vi "CRYextision level.vi"(6 "measured SPL":dbl[](array[numeric]), 7 "measured frequency":dbl[](array[numeric])) -> (5 "extition level":dbl[](array[numeric]))   [LabVIEW 2013]
panel:
  out "extition level 2":dbl[](array[numeric])
  out "repeated nuber":dbl[](array[numeric])
  in  "delta":dbl[](array[numeric])
  in  "fixed frequency":dbl[](array[numeric])
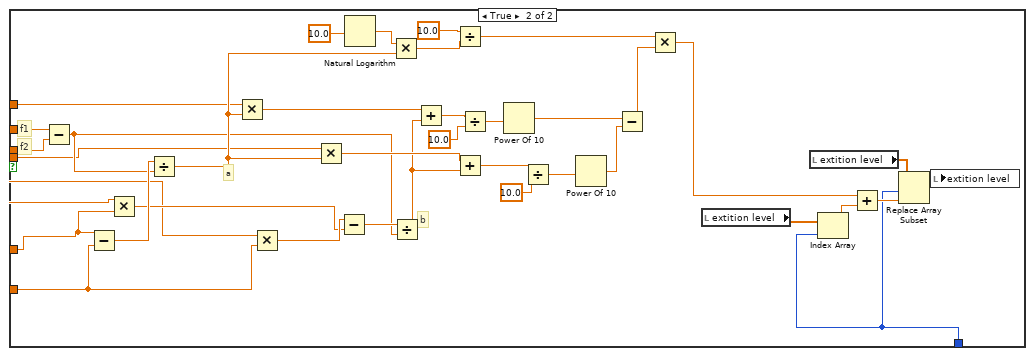
[diagram p4: hidden frame]
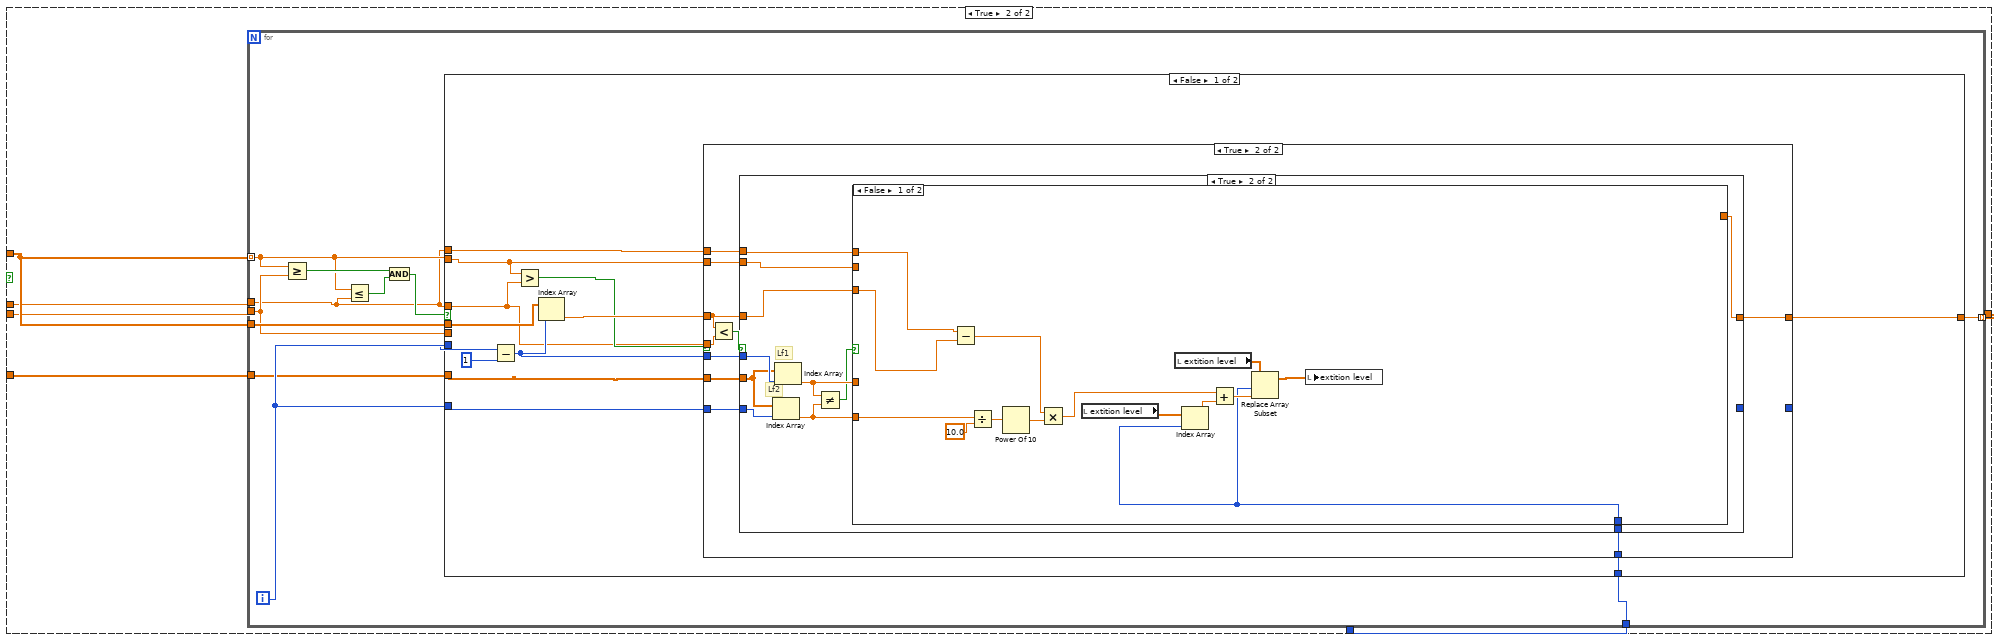
[diagram p5: hidden frame]
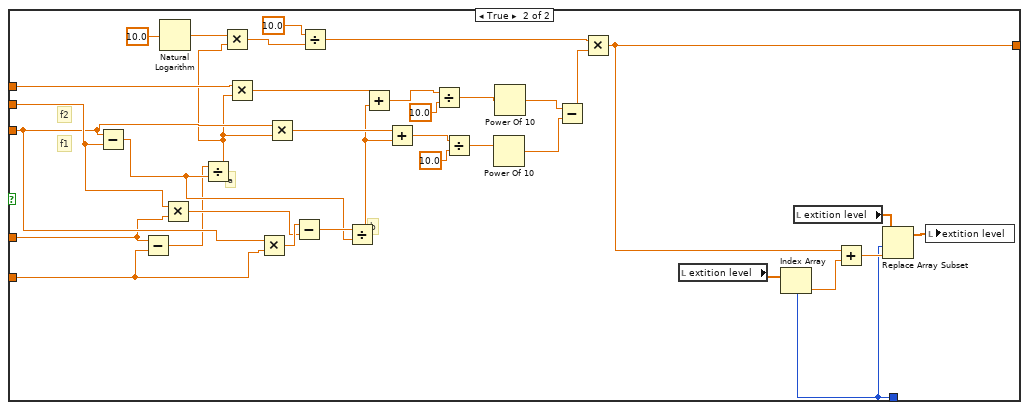
[diagram p8: hidden frame]
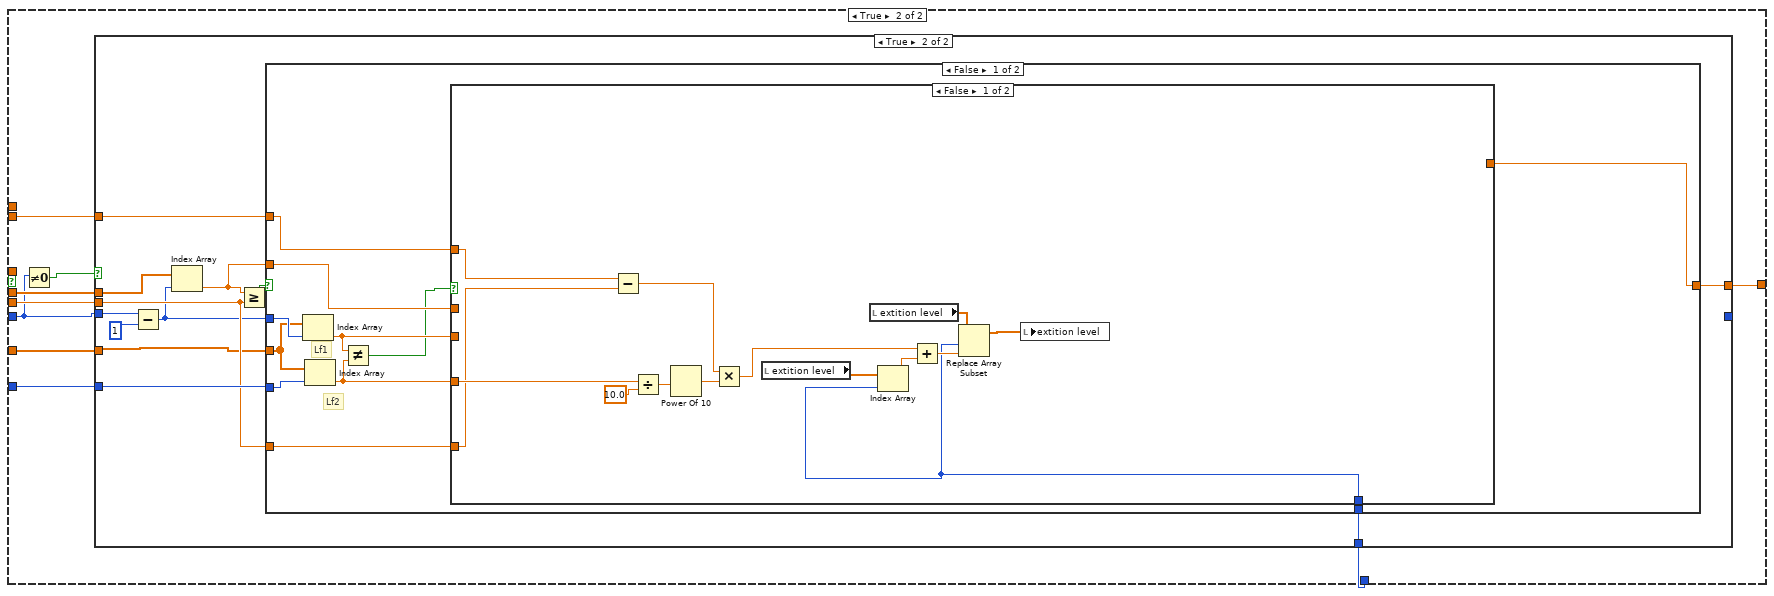
[diagram p9: hidden frame]
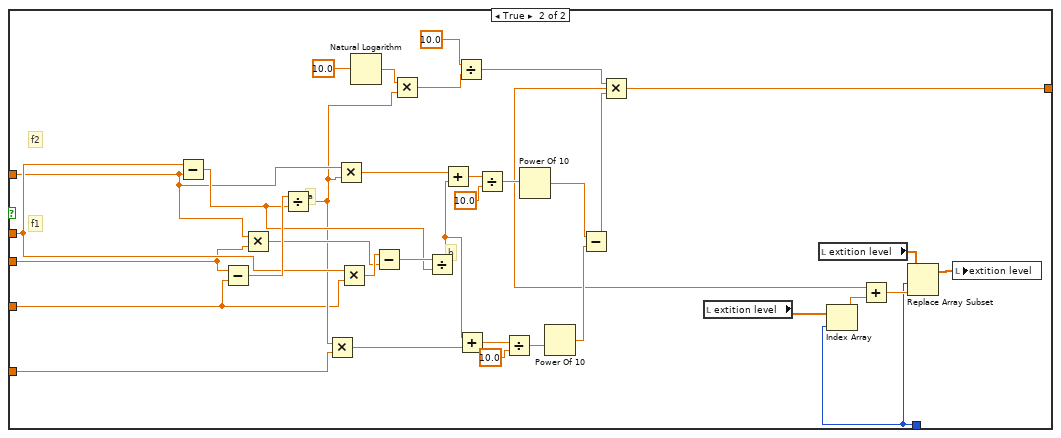
[diagram p11: hidden frame]
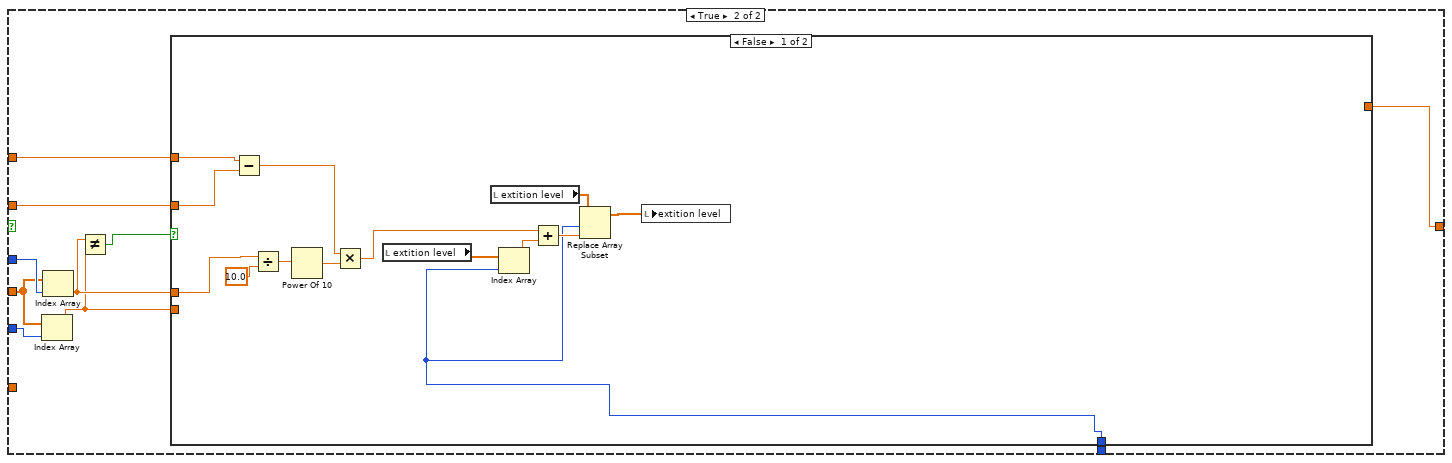
[diagram p12: hidden frame]
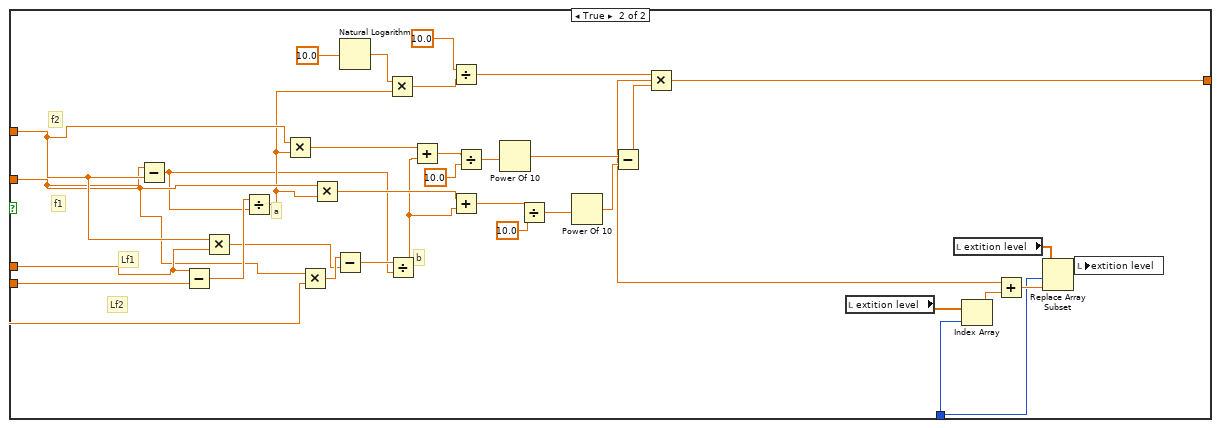
[diagram p13: hidden frame]
diagram:
  n1 = flat-sequence {
    tunnel: [w5] -> w2
    frame #0 {
      n2 = Initialize Array(0.0, 29) -> (w5:dbl[])
      n3 = local write "repeated nuber"(w5) -> ()
      n4 = local write "fixed frequency"(dbl[] [20.0, 25.0, 31.5, 40.0, 50.0, 63.0, 80.0, 100.0, 125.0, 160.0, 200.0, 267.0, 339.0, 436.0, 552.0, 707.7, 899.5, 1112.0, 1406.0, 1827.58, 2288.5, 2813.46, 3501.8, 4289.16, 5099.67, 6148.1, 7303.7, 8309.5, 9452.87, 15500.0]) -> ()
      n5 = local write "extition level"(w5) -> ()
      n6 = local write "delta"(dbl[] [5.0, 6.5, 8.5, 10.0, 13.0, 17.0, 20.0, 25.0, 35.0, 40.0, 67.0, 72.0, 97.0, 116.0, 155.7, 191.8, 202.5, 294.0, 421.58, 460.9, 524.9, 688.3, 787.3, 810.5, 1048.4, 1155.6, 1005.8, 1143.37, 6047.13]) -> ()
    }
  }
  n7 = flat-sequence {
    tunnel: w2 -> [_]
    tunnel: [w8] -> w1
    frame #0 {
      n8 = local read "measured frequency"() -> (w9:dbl[])
      n9 = local read "fixed frequency"() -> (w10:dbl[])
      n10 = for {
        tunnel: w10 -> [w17] mode=indexing
        tunnel: w9 -> [w18]
        tunnel: w10 -> [w16]
        tunnel: [w11] -> w8 mode=indexing
        i -> [w12]
        n11 = Add(x=1.0, y=w12) -> (x+y=w14:dbl)
        n12 = Index Array(array=w16, index=w14) -> (element=w13:dbl)
        n13 = for {
          tunnel: w18 -> [w19] mode=indexing
          tunnel: w17 -> [w26]
          tunnel: w13 -> [w20]
          tunnel: w12 -> [w22]
          tunnel: [w21] -> w11 mode=indexing
          n14 = Greater Or Equal?(x=w19, y=w26) -> (x >= y?=w24:bool)
          n15 = Less Or Equal?(x=w19, y=w20) -> (x <= y?=w25:bool)
          n16 = And(x=w25, y=w24) -> (x .and. y?=w23:bool)
          n17 = case shown="True" w23 {
            tunnel: w22 -> [w27 w31]
            tunnel: [w27 _] -> w21
            frame False {
            }
            frame True {
              n18 = local read "repeated nuber"() -> (w32:dbl[])
              n19 = local read "repeated nuber"() -> (w34:dbl[])
              n20 = Index Array(array=w32, index=w31) -> (element=w30:dbl)
              n21 = Add(x=1.0, y=w30) -> (x+y=w28:dbl)
              n22 = Replace Array Subset(array=w34, new element=w28, index=w31) -> (w33:dbl[])
              n23 = local write "repeated nuber"(w33) -> ()
            }
          }
        }
      }
    }
  }
  n24 = flat-sequence {
    tunnel: w1 -> [_]
    frame #0 {
      n25 = local read "measured frequency"() -> (w36:dbl[])
      n26 = local read "fixed frequency"() -> (w37:dbl[])
      n27 = local read "repeated nuber"() -> (w39:dbl[])
      n28 = local read "measured SPL"() -> (w35:dbl[])
      n29 = local read "delta"() -> (w38:dbl[])
      n30 = for {
        tunnel: w39 -> [w45] mode=indexing
        tunnel: w37 -> [w50] mode=indexing
        tunnel: w38 -> [w41] mode=indexing
        tunnel: w37 -> [w49]
        tunnel: w36 -> [w44]
        tunnel: w35 -> [w43]
        i -> [w40]
        n31 = Add(x=w40, y=1) -> (x+y=w46:i32)
        n32 = Index Array(array=w49, index=w46) -> (element=w48:dbl)
        n33 = Not Equal To 0?(x=w45) -> (x != 0?=w51:bool)
        n34 = case shown="False" w51 {
          tunnel: w44 -> [w66 w147]
          tunnel: w50 -> [w64 w146]
          tunnel: w43 -> [w65 w145]
          tunnel: w48 -> [w63 w144]
          tunnel: [_ w143] -> w42
          tunnel: w40 -> [w62 w142]
          frame False {
            n35 = for {
              tunnel: w66 -> [w74] mode=indexing
              tunnel: w64 -> [w68]
              tunnel: w66 -> [w79]
              tunnel: w65 -> [w73]
              tunnel: w63 -> [w70]
              tunnel: w62 -> [w69]
              tunnel: w63 -> [w67]
              i -> [w71]
              n36 = Add(x=1, y=w71) -> (x+y=w72:i32)
              n37 = Less?(x=w74, y=w68) -> (x < y?=w78:bool)
              n38 = Index Array(array=w79, index=w72) -> (element=w75:dbl)
              n39 = Greater?(x=w75, y=w67) -> (0:w77:bool)
              n40 = And(x=w78, y=w77) -> (x .and. y?=w76:bool)
              n41 = case shown="True" w76 {
                tunnel: w75 -> [_ w91]
                tunnel: w74 -> [_ w85]
                tunnel: w73 -> [_ w90]
                tunnel: w72 -> [_ w89]
                tunnel: w71 -> [_ w88]
                tunnel: w70 -> [_ w87]
                tunnel: w69 -> [_ w86]
                tunnel: w68 -> [_ w84]
                frame False {
                }
                frame True {
                  # "Lf2"
                  # "Lf1"
                  n42 = Index Array(array=w90, index=w88) -> (element=w83:dbl)
                  n43 = Index Array(array=w90, index=w89) -> (element=w82:dbl)
                  n44 = Not Equal?(x=w83, y=w82) -> (x != y?=w81:bool)
                  n45 = case shown="False" w81 {
                    tunnel: w91 -> [_ w113]
                    tunnel: w87 -> [w94 w112]
                    tunnel: w86 -> [w92 w111]
                    tunnel: w85 -> [_ w110]
                    tunnel: w84 -> [w93 w109]
                    tunnel: w83 -> [w95 w107]
                    tunnel: w82 -> [_ w106]
                    frame False {
                      n46 = Subtract(x=w94, y=w93) -> (x-y=w102:dbl)
                      n47 = Divide(x=w95, y=10.0) -> (x/y=w104:dbl)
                      n48 = Power Of 10(x=w104) -> (10^x=w103:dbl)
                      n49 = Multiply(x=w102, y=w103) -> (x*y=w96:dbl)
                      n50 = local read "extition level"() -> (w100:dbl[])
                      n51 = local read "extition level"() -> (w101:dbl[])
                      n52 = Index Array(array=w100, index=w92) -> (element=w99:dbl)
                      n53 = Add(x=w96, y=w99) -> (x+y=w98:dbl)
                      n54 = Replace Array Subset(array=w101, new element=w98, index=w92) -> (w97:dbl[])
                      n55 = local write "extition level"(w97) -> ()
                    }
                    frame True {
                      # "b"
                      # "a"
                      # "f2"
                      # "f1"
                      n56 = Subtract(x=w110, y=w113) -> (x-y=w114:dbl)
                      n57 = Subtract(x=w107, y=w106) -> (x-y=w141:dbl)
                      n58 = Multiply(x=w113, y=w107) -> (x*y=w139:dbl)
                      n59 = Divide(x=w141, y=w114) -> (x/y=w119:dbl)
                      n60 = Multiply(x=w112, y=w119) -> (x*y=w132:dbl)
                      n61 = Multiply(x=w110, y=w106) -> (x*y=w140:dbl)
                      n62 = Multiply(x=w109, y=w119) -> (x*y=w128:dbl)
                      n63 = Subtract(x=w140, y=w139) -> (x-y=w138:dbl)
                      n64 = Natural Logarithm(1:10.0) -> (0:w120:dbl)
                      n65 = Multiply(x=w120, y=w119) -> (x*y=w118:dbl)
                      n66 = Divide(x=w138, y=w114) -> (x/y=w127:dbl)
                      n67 = Add(x=w132, y=w127) -> (x+y=w131:dbl)
                      n68 = Divide(x=10.0, y=w118) -> (x/y=w116:dbl)
                      n69 = Add(x=w128, y=w127) -> (x+y=w124:dbl)
                      n70 = Divide(x=w131, y=10.0) -> (x/y=w129:dbl)
                      n71 = Power Of 10(x=w129) -> (10^x=w123:dbl)
                      n72 = Divide(x=w124, y=10.0) -> (x/y=w126:dbl)
                      n73 = Power Of 10(x=w126) -> (10^x=w122:dbl)
                      n74 = Subtract(x=w123, y=w122) -> (x-y=w115:dbl)
                      n75 = Multiply(x=w116, y=w115) -> (x*y=w108:dbl)
                      n76 = local read "extition level"() -> (w135:dbl[])
                      n77 = local read "extition level"() -> (w136:dbl[])
                      n78 = Index Array(array=w135, index=w111) -> (element=w134:dbl)
                      n79 = Add(x=w108, y=w134) -> (x+y=w133:dbl)
                      n80 = Replace Array Subset(array=w136, new element=w133, index=w111) -> (w137:dbl[])
                      n81 = local write "extition level"(w137) -> ()
                    }
                  }
                }
              }
            }
          }
          frame True {
            n82 = for {
              tunnel: w147 -> [w152] mode=indexing
              tunnel: w146 -> [w153]
              tunnel: w147 -> [w155]
              tunnel: w145 -> [w150]
              tunnel: w142 -> [w154]
              tunnel: [w149] -> w143 mode=indexing
              tunnel: w144 -> [w148]
              i -> [w151]
              n83 = Greater Or Equal?(x=w152, y=w153) -> (x >= y?=w157:bool)
              n84 = Less Or Equal?(x=w152, y=w148) -> (x <= y?=w158:bool)
              n85 = And(x=w157, y=w158) -> (x .and. y?=w156:bool)
              n86 = case shown="False" w156 {
                tunnel: w151 -> [w170 w245]
                tunnel: w155 -> [w171 w247]
                tunnel: w153 -> [_ w248]
                tunnel: w150 -> [w162 w252]
                tunnel: w151 -> [w168 w251]
                tunnel: w152 -> [w161 w250]
                tunnel: w154 -> [w166 w249]
                tunnel: w148 -> [w167 _]
                tunnel: w148 -> [w159 _]
                tunnel: [w163 w244] -> w149
                frame False {
                  n87 = Subtract(x=w170, y=1) -> (x-y=w169:i32)
                  n88 = Greater?(x=w161, y=w159) -> (0:w160:bool)
                  n89 = Index Array(array=w171, index=w169) -> (element=w164:dbl)
                  n90 = case shown="True" w160 {
                    tunnel: w169 -> [_ w182]
                    tunnel: w168 -> [w172 w181]
                    tunnel: w167 -> [_ w180]
                    tunnel: w166 -> [_ w179]
                    tunnel: w164 -> [_ w174]
                    tunnel: [_ w178] -> w163
                    tunnel: w162 -> [_ w177]
                    tunnel: w161 -> [_ w176]
                    tunnel: w159 -> [_ w175]
                    tunnel: [w172 _] -> _
                    frame False {
                    }
                    frame True {
                      n91 = Less?(x=w174, y=w175) -> (x < y?=w173:bool)
                      n92 = case shown="True" w173 {
                        tunnel: w176 -> [_ w194]
                        tunnel: w177 -> [_ w190]
                        tunnel: w182 -> [_ w193]
                        tunnel: w181 -> [w183 w192]
                        tunnel: w180 -> [_ w189]
                        tunnel: w179 -> [_ w191]
                        tunnel: w174 -> [_ w188]
                        tunnel: [_ w187] -> w178
                        tunnel: [w183 _] -> _
                        frame False {
                        }
                        frame True {
                          # "Lf2"
                          # "Lf1"
                          n93 = Index Array(array=w190, index=w192) -> (element=w185:dbl)
                          n94 = Index Array(array=w190, index=w193) -> (element=w186:dbl)
                          n95 = Not Equal?(x=w186, y=w185) -> (x != y?=w184:bool)
                          n96 = case shown="False" w184 {
                            tunnel: w194 -> [_ w237]
                            tunnel: w191 -> [w195 w236]
                            tunnel: w189 -> [w197 w233]
                            tunnel: w188 -> [w196 w231]
                            tunnel: [_ w211] -> w187
                            tunnel: w186 -> [_ w210]
                            tunnel: w185 -> [w198 w209]
                            frame False {
                              n97 = Subtract(x=w197, y=w196) -> (x-y=w205:dbl)
                              n98 = Divide(x=w198, y=10.0) -> (x/y=w207:dbl)
                              n99 = Power Of 10(x=w207) -> (10^x=w206:dbl)
                              n100 = Multiply(x=w205, y=w206) -> (x*y=w199:dbl)
                              n101 = local read "extition level"() -> (w203:dbl[])
                              n102 = local read "extition level"() -> (w204:dbl[])
                              n103 = Index Array(array=w203, index=w195) -> (element=w202:dbl)
                              n104 = Add(x=w199, y=w202) -> (x+y=w201:dbl)
                              n105 = Replace Array Subset(array=w204, new element=w201, index=w195) -> (w200:dbl[])
                              n106 = local write "extition level"(w200) -> ()
                            }
                            frame True {
                              # "b"
                              # "a"
                              # "f2"
                              # "f1"
                              n107 = Subtract(x=w231, y=w237) -> (x-y=w235:dbl)
                              n108 = Subtract(x=w210, y=w209) -> (x-y=w228:dbl)
                              n109 = Natural Logarithm(1:10.0) -> (0:w217:dbl)
                              n110 = Multiply(x=w237, y=w210) -> (x*y=w242:dbl)
                              n111 = Divide(x=w228, y=w235) -> (x/y=w219:dbl)
                              n112 = Multiply(x=w217, y=w219) -> (x*y=w215:dbl)
                              n113 = Multiply(x=w233, y=w219) -> (x*y=w232:dbl)
                              n114 = Multiply(x=w231, y=w209) -> (x*y=w243:dbl)
                              n115 = Multiply(x=w231, y=w219) -> (x*y=w230:dbl)
                              n116 = Subtract(x=w243, y=w242) -> (x-y=w241:dbl)
                              n117 = Divide(x=10.0, y=w215) -> (x/y=w214:dbl)
                              n118 = Divide(x=w241, y=w235) -> (x/y=w229:dbl)
                              n119 = Add(x=w232, y=w229) -> (x+y=w227:dbl)
                              n120 = Add(x=w230, y=w229) -> (x+y=w224:dbl)
                              n121 = Divide(x=w227, y=10.0) -> (x/y=w223:dbl)
                              n122 = Divide(x=w224, y=10.0) -> (x/y=w222:dbl)
                              n123 = Power Of 10(x=w222) -> (10^x=w220:dbl)
                              n124 = Power Of 10(x=w223) -> (10^x=w221:dbl)
                              n125 = Subtract(x=w221, y=w220) -> (x-y=w213:dbl)
                              n126 = Multiply(x=w214, y=w213) -> (x*y=w211:dbl)
                              n127 = local read "extition level"() -> (w212:dbl[])
                              n128 = Index Array(array=w212, index=w236) -> (element=w239:dbl)
                              n129 = local read "extition level"() -> (w240:dbl[])
                              n130 = Add(x=w211, y=w239) -> (x+y=w238:dbl)
                              n131 = Replace Array Subset(array=w240, new element=w238, index=w236) -> (w234:dbl[])
                              n132 = local write "extition level"(w234) -> ()
                            }
                          }
                        }
                      }
                    }
                  }
                }
                frame True {
                  n133 = Not Equal To 0?(x=w245) -> (x != 0?=w246:bool)
                  n134 = case shown="True" w246 {
                    tunnel: w245 -> [w253 w256]
                    tunnel: w252 -> [_ w254]
                    tunnel: w251 -> [_ w265]
                    tunnel: w250 -> [_ w264]
                    tunnel: w249 -> [_ w263]
                    tunnel: w248 -> [_ w262]
                    tunnel: w247 -> [_ w261]
                    tunnel: [_ w255] -> w244
                    tunnel: [w253 _] -> _
                    frame False {
                    }
                    frame True {
                      n135 = Subtract(x=w256, y=1) -> (x-y=w258:i32)
                      n136 = Index Array(array=w261, index=w258) -> (element=w257:dbl)
                      n137 = Greater Or Equal?(x=w257, y=w262) -> (x >= y?=w259:bool)
                      n138 = case shown="False" w259 {
                        tunnel: w254 -> [w275 w332]
                        tunnel: w258 -> [w276 w335]
                        tunnel: w265 -> [w274 w334]
                        tunnel: w257 -> [w273 w330]
                        tunnel: w264 -> [w271 w331]
                        tunnel: w263 -> [w272 w333]
                        tunnel: w262 -> [w270 _]
                        tunnel: [w269 w329] -> w255
                        frame False {
                          # "Lf2"
                          # "Lf1"
                          n139 = Index Array(array=w275, index=w276) -> (element=w268:dbl)
                          n140 = Index Array(array=w275, index=w274) -> (element=w267:dbl)
                          n141 = Not Equal?(x=w268, y=w267) -> (x != y?=w266:bool)
                          n142 = case shown="False" w266 {
                            tunnel: w273 -> [_ w317]
                            tunnel: w272 -> [w277 w315]
                            tunnel: w271 -> [w279 w313]
                            tunnel: w270 -> [w278 w308]
                            tunnel: [_ w293] -> w269
                            tunnel: w268 -> [_ w292]
                            tunnel: w267 -> [w280 w291]
                            frame False {
                              n143 = Subtract(x=w279, y=w278) -> (x-y=w287:dbl)
                              n144 = Divide(x=w280, y=10.0) -> (x/y=w289:dbl)
                              n145 = Power Of 10(x=w289) -> (10^x=w288:dbl)
                              n146 = Multiply(x=w287, y=w288) -> (x*y=w281:dbl)
                              n147 = local read "extition level"() -> (w285:dbl[])
                              n148 = local read "extition level"() -> (w286:dbl[])
                              n149 = Index Array(array=w285, index=w277) -> (element=w284:dbl)
                              n150 = Add(x=w281, y=w284) -> (x+y=w283:dbl)
                              n151 = Replace Array Subset(array=w286, new element=w283, index=w277) -> (w282:dbl[])
                              n152 = local write "extition level"(w282) -> ()
                            }
                            frame True {
                              # "b"
                              # "a"
                              # "f2"
                              # "f1"
                              n153 = Subtract(x=w317, y=w313) -> (x-y=w321:dbl)
                              n154 = Subtract(x=w292, y=w291) -> (x-y=w325:dbl)
                              n155 = Multiply(x=w313, y=w292) -> (x*y=w323:dbl)
                              n156 = Divide(x=w325, y=w321) -> (x/y=w298:dbl)
                              n157 = Multiply(x=w298, y=w308) -> (x*y=w307:dbl)
                              n158 = Multiply(x=w313, y=w298) -> (x*y=w312:dbl)
                              n159 = Multiply(x=w317, y=w291) -> (x*y=w324:dbl)
                              n160 = Natural Logarithm(1:10.0) -> (0:w299:dbl)
                              n161 = Subtract(x=w324, y=w323) -> (x-y=w322:dbl)
                              n162 = Multiply(x=w299, y=w298) -> (x*y=w296:dbl)
                              n163 = Divide(x=w322, y=w321) -> (x/y=w306:dbl)
                              n164 = Add(x=w312, y=w306) -> (x+y=w311:dbl)
                              n165 = Divide(x=10.0, y=w296) -> (x/y=w295:dbl)
                              n166 = Add(x=w306, y=w307) -> (x+y=w304:dbl)
                              n167 = Divide(x=w311, y=10.0) -> (x/y=w309:dbl)
                              n168 = Divide(x=w304, y=10.0) -> (x/y=w305:dbl)
                              n169 = Power Of 10(x=w309) -> (10^x=w302:dbl)
                              n170 = Power Of 10(x=w305) -> (10^x=w301:dbl)
                              n171 = Subtract(x=w302, y=w301) -> (x-y=w294:dbl)
                              n172 = Multiply(x=w295, y=w294) -> (x*y=w293:dbl)
                              n173 = local read "extition level"() -> (w319:dbl[])
                              n174 = local read "extition level"() -> (w320:dbl[])
                              n175 = Index Array(array=w319, index=w315) -> (element=w318:dbl)
                              n176 = Add(x=w293, y=w318) -> (x+y=w316:dbl)
                              n177 = Replace Array Subset(array=w320, new element=w316, index=w315) -> (w314:dbl[])
                              n178 = local write "extition level"(w314) -> ()
                            }
                          }
                        }
                        frame True {
                          n179 = Index Array(array=w332, index=w334) -> (element=w326:dbl)
                          n180 = Index Array(array=w332, index=w335) -> (element=w327:dbl)
                          n181 = Not Equal?(x=w327, y=w326) -> (x != y?=w328:bool)
                          n182 = case shown="False" w328 {
                            tunnel: w326 -> [_ w382]
                            tunnel: w327 -> [w349 w381]
                            tunnel: w333 -> [w336 w373]
                            tunnel: w331 -> [w346 w368]
                            tunnel: w330 -> [w345 w367]
                            tunnel: [_ w350] -> w329
                            frame False {
                              n183 = Subtract(x=w346, y=w345) -> (x-y=w343:dbl)
                              n184 = Divide(x=w349, y=10.0) -> (x/y=w347:dbl)
                              n185 = Power Of 10(x=w347) -> (10^x=w344:dbl)
                              n186 = Multiply(x=w343, y=w344) -> (x*y=w337:dbl)
                              n187 = local read "extition level"() -> (w341:dbl[])
                              n188 = local read "extition level"() -> (w342:dbl[])
                              n189 = Index Array(array=w341, index=w336) -> (element=w340:dbl)
                              n190 = Add(x=w337, y=w340) -> (x+y=w339:dbl)
                              n191 = Replace Array Subset(array=w342, new element=w339, index=w336) -> (w338:dbl[])
                              n192 = local write "extition level"(w338) -> ()
                            }
                            frame True {
                              # "b"
                              # "a"
                              # "f2"
                              # "f1"
                              # "Lf2"
                              # "Lf1"
                              n193 = Subtract(x=w367, y=w368) -> (x-y=w351:dbl)
                              n194 = Subtract(x=w381, y=w382) -> (x-y=w383:dbl)
                              n195 = Multiply(x=w368, y=w381) -> (x*y=w379:dbl)
                              n196 = Divide(x=w383, y=w351) -> (x/y=w357:dbl)
                              n197 = Multiply(x=w368, y=w357) -> (x*y=w372:dbl)
                              n198 = Multiply(x=w367, y=w382) -> (x*y=w380:dbl)
                              n199 = Multiply(x=w367, y=w357) -> (x*y=w366:dbl)
                              n200 = Subtract(x=w380, y=w379) -> (x-y=w378:dbl)
                              n201 = Natural Logarithm(1:10.0) -> (0:w358:dbl)
                              n202 = Multiply(x=w358, y=w357) -> (x*y=w356:dbl)
                              n203 = Divide(x=w378, y=w351) -> (x/y=w365:dbl)
                              n204 = Add(x=w372, y=w365) -> (x+y=w371:dbl)
                              n205 = Divide(x=10.0, y=w356) -> (x/y=w354:dbl)
                              n206 = Add(x=w366, y=w365) -> (x+y=w362:dbl)
                              n207 = Divide(x=w371, y=10.0) -> (x/y=w369:dbl)
                              n208 = Power Of 10(x=w369) -> (10^x=w361:dbl)
                              n209 = Divide(x=w362, y=10.0) -> (x/y=w364:dbl)
                              n210 = Power Of 10(x=w364) -> (10^x=w360:dbl)
                              n211 = Subtract(x=w361, y=w360) -> (x-y=w353:dbl)
                              n212 = Multiply(x=w354, y=w353) -> (x*y=w350:dbl)
                              n213 = local read "extition level"() -> (w352:dbl[])
                              n214 = local read "extition level"() -> (w376:dbl[])
                              n215 = Index Array(array=w352, index=w373) -> (element=w375:dbl)
                              n216 = Add(x=w350, y=w375) -> (x+y=w374:dbl)
                              n217 = Replace Array Subset(array=w376, new element=w374, index=w373) -> (w377:dbl[])
                              n218 = local write "extition level"(w377) -> ()
                            }
                          }
                        }
                      }
                    }
                  }
                }
              }
            }
          }
        }
        n219 = flat-sequence {
          tunnel: w41 -> [w61]
          tunnel: w40 -> [w53]
          tunnel: w42 -> [_]
          frame #0 {
            n220 = local read "extition level"() -> (w54:dbl[])
            n221 = local read "extition level"() -> (w60:dbl[])
            n222 = Index Array(array=w54, index=w53) -> (element=w59:dbl)
            n223 = Divide(x=w59, y=w61) -> (x/y=w56:dbl)
            n224 = Logarithm Base 10(1:w56) -> (0:w57:dbl)
            n225 = Multiply(x=w57, y=10.0) -> (x*y=w55:dbl)
            n226 = Replace Array Subset(array=w60, new element=w55, index=w53) -> (w52:dbl[])
            n227 = local write "extition level"(w52) -> ()
          }
        }
      }
    }
  }
